vi "CreateNewWizard_Invoke Core.vi"(6 "what to make":T1, 10 "Wizard":T3, 11 "Cluster":T2) -> (3 "Canceled":bool)   [LabVIEW 2020, in "Add Actor.lvlib"]
uses:
  Add Actor.lvlib
  <resource>/Framework/Providers/API/ItemRef.ctl
  <resource>/Framework/Providers/API/mxLvNIIM.ctl
  What To Make.ctl
  Localized Strings.vi
  AddActorInterface/Add Actor Interface.lvlib
  MessageMakerProvider/AFPP Shared/AFPP Shared.lvlib
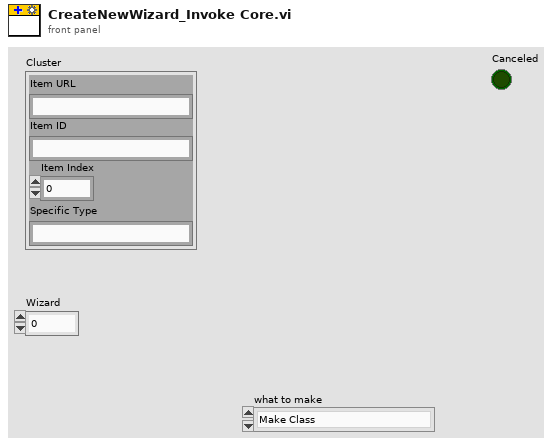
[diagram p1: front panel]
types:
  T1 = typedef "Add Actor.lvlib/What To Make.ctl" = enum16{"Make Class", "Make Interface"}
  T2 = typedef "mxLvNIIM.ctl" = cluster{"Item URL":string, "Item ID":string, "Item Index":i32, "Specific Type":string}
  T3 = typedef "ItemRef.ctl" = u64
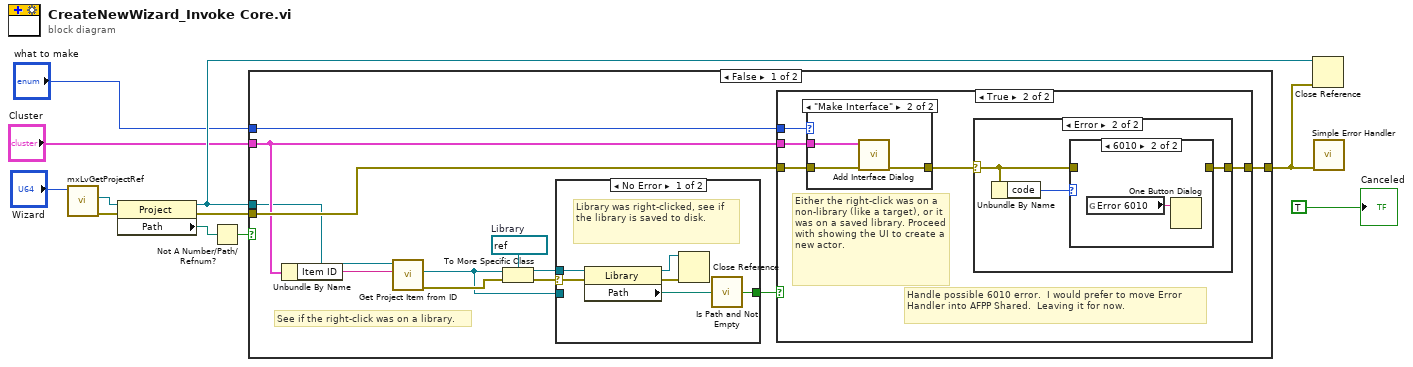
[diagram p0: block diagram]
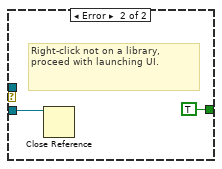
[diagram p2: hidden frame]
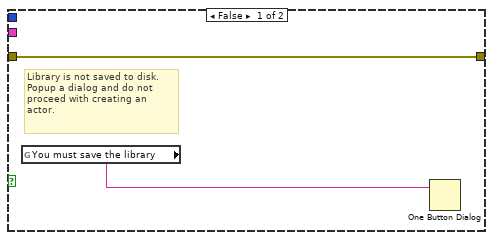
[diagram p3: hidden frame]
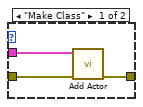
[diagram p4: hidden frame]
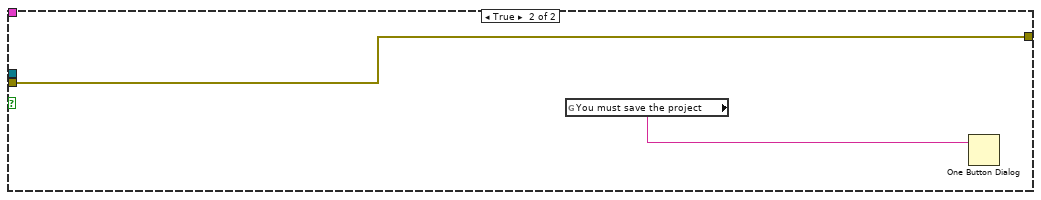
[diagram p7: hidden frame]
diagram:
  n1 = call <resource>:"mxLvGetProjectRef.vi"("Item"="Wizard") -> ("error out"=w5:errorcluster, "Project Refnum"=w4:refnum<vi>)  [unwired: 8 in, 1 out]
  n2 = property class="Project"(reference=w4, error in=w5) -> (reference out=w11:refnum<vi>, error out=w8:errorcluster, "Path"=w6:path)
  n3 = Not A Number/Path/Refnum?(number/path/refnum=w6) -> (NaN/Path/Refnum?=w7:bool)
  n4 = case shown="False" w7 {
    tunnel: [w23 w52] -> w10
    tunnel: "Cluster" -> [w17 _]
    tunnel: w8 -> [w22 w52]
    tunnel: w11 -> [w15 _]
    tunnel: "what to make" -> [w16 _]
    frame False {
      w21 = refnum<vi> refnum  # Library
      # "See if the right-click was on a library."
      n5 = Unbundle By Name(w17) -> ("Item ID"=w14:string)
      n6 = call "Get Project Item from ID.vi"("Item ID"=w14, "Project in"=w15) -> ("error out"=w13:errorcluster, "Project Item"=w12:refnum<vi>)  [unwired: 7 in, 1 out]
      n7 = To More Specific Class(target class=w21, reference=w12, error in=w13) -> (specific class reference=w20:refnum<vi>, error out=w19:errorcluster)
      n8 = case shown="No Error" w19 {
        selector: w19 -> [w28 _]
        tunnel: w20 -> [w29 _]
        tunnel: [w24 TRUE ("Is Path and Not Empty?")] -> w18
        tunnel: w12 -> [_ w30]
        frame No Error {
          # "Library was right-clicked, see if the library is saved to disk."
          n9 = property class="Library"(reference=w29, error in=w28) -> (reference out=w26:refnum<vi>, error out=w27:errorcluster, "Path"=w25:path)
          n10 = Close Reference(reference=w26, error in (no error)=w27) -> ()  [unwired: 1 out]
          n11 = call <vilib>:"Is Path and Not Empty.vi"("path"=w25) -> ("Is Path and Not Empty?"=w24:bool)  [unwired: 4 in]
        }
        frame Error {
          # "Right-click not on a library, proceed with launching UI."
          n12 = Close Reference(reference=w30) -> ()  [unwired: 1 in, 1 out]
        }
      }
      n13 = case shown="True" w18 {
        tunnel: [w33 w35] -> w23
        tunnel: w17 -> [_ w38]
        tunnel: w22 -> [w33 w37]
        tunnel: w16 -> [_ w34]
        frame False {
          # "Library is not saved to disk. Popup a dialog and do not proceed with creating an actor."
          n14 = global read "Localized Strings.vi" "You must save the library"() -> (w32:string)
          n15 = One Button Dialog(message=w32) -> ()  [unwired: 1 in, 1 out]
        }
        frame True {
          # "Handle possible 6010 error.  I would prefer to move Error Handler into AFPP Shared.  Leaving it for now."
          # "Either the right-click was on a non-library (like a target), or it was on a saved library. Proceed with showing the UI to create a new actor."
          n16 = case shown="\"Make Interface\"" w34 {
            tunnel: w38 -> [w41 w42]
            tunnel: w37 -> [w40 w44]
            tunnel: [w39 w43] -> w36
            frame "Make Class" {
              n17 = call "Add Actor.vi"("error in"=w40, "Target Item"=w41) -> ("error out"=w39:errorcluster)  [unwired: 9 in]
            }
            frame "Make Interface" {
              n18 = call "Add Interface Dialog.vi"("error in"=w44, "Target Item"=w42) -> ("error out"=w43:errorcluster)  [unwired: 9 in]
            }
          }
          n19 = case shown="Error" w36 {
            selector: w36 -> [w45 w46]
            tunnel: [w45 w48] -> w35
            frame No Error {
            }
            frame Error {
              n20 = Unbundle By Name(w46) -> ("code"=w47:i32)
              n21 = case shown="6010" w47 {
                tunnel: [w49 _] -> w48
                tunnel: w46 -> [w49 _]
                frame Default {
                }
                frame 6010 {
                  n22 = global read "Localized Strings.vi" "Error 6010"() -> (w50:string)
                  n23 = One Button Dialog(message=w50) -> ()  [unwired: 1 in, 1 out]
                }
              }
            }
          }
        }
      }
    }
    frame True {
      n24 = global read "Localized Strings.vi" "You must save the project"() -> (w51:string)
      n25 = One Button Dialog(message=w51) -> ()  [unwired: 1 in, 1 out]
    }
  }
  n26 = Close Reference(reference=w11, error in (no error)=w10) -> ()  [unwired: 1 out]
  n27 = call <vilib>:"Simple Error Handler.vi"("error in (no error)"=w10) -> ()  [unwired: 4 in, 5 out]
  "Canceled" <- TRUE ("Canceled")
